vi "Cal_Gain&offset.vi"(7 "REAL2":dbl, 8 "REAL1":dbl, 9 "AD2":dbl, 10 "AD1":dbl) -> (2 "Offset":i32 format="%x", 3 "Gain":dbl)   [LabVIEW 2013]
panel:
  out "x-y":i32 format="%x"
  out "Offset":i32 format="%x"
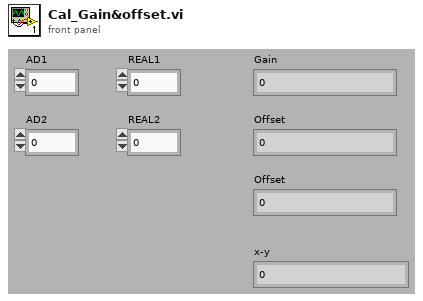
[diagram p1: front panel]
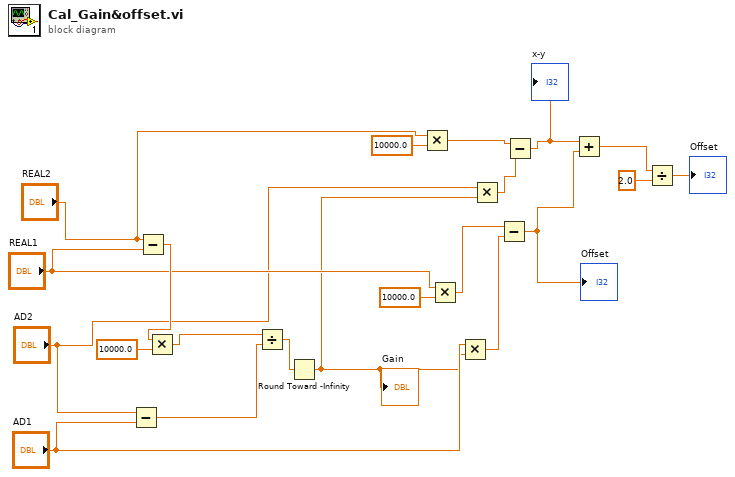
[diagram p0: block diagram]
diagram:
  n1 = Subtract(x="AD2", y="AD1") -> (x-y=w9:dbl)
  n2 = Subtract(x="REAL2", y="REAL1") -> (x-y=w20:dbl)
  n3 = Multiply(x=w20, y=10000.0) -> (x*y=w19:dbl)
  n4 = Divide(x=w19, y=w9) -> (x/y=w2:dbl)
  n5 = Round Toward -Infinity(1:w2) -> (0:w1:dbl)
  "Gain" <- w1
  n6 = Multiply(x="REAL2", y=10000.0) -> (x*y=w11:dbl)
  n7 = Multiply(x="REAL1", y=10000.0) -> (x*y=w16:dbl)
  n8 = Multiply(x="AD1", y=w1) -> (x*y=w14:dbl)
  n9 = Multiply(x="AD2", y=w1) -> (x*y=w10:dbl)
  n10 = Subtract(x=w16, y=w14) -> (x-y=w7:dbl)
  "Offset" <- w7
  n11 = Subtract(x=w11, y=w10) -> (x-y=w8:dbl)
  "x-y" <- w8
  n12 = Add(x=w8, y=w7) -> (x+y=w6:dbl)
  n13 = Divide(x=w6, y=2.0) -> (x/y=→"Offset":dbl)
